vi "1part.vi"(3 "Кол-во бит":i32) -> (1 "Вырезка из массива":dbl[](array[numeric]))   [LabVIEW 2017]
panel:
  in  "Сколько битов брать":i32=4
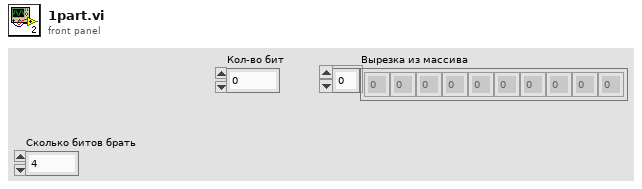
[diagram p1: front panel]
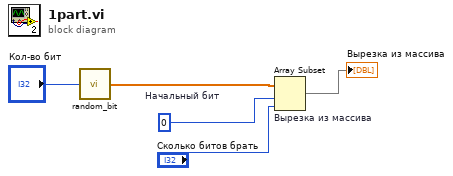
[diagram p0: block diagram]
diagram:
  w4 = 0  # Начальный бит
  n1 = call "random_bit.vi"("Количество бит"="Кол-во бит") -> ("Биты на выходе 1"=w2:dbl[])
  n2 = Array Subset "Вырезка из массива"(array=w2, index=w4, length="Сколько битов брать") -> (→"Вырезка из массива":dbl[])
